vi "SMTP Email Alerts Engine.vi"(0 "Notifier Name":string, 11 "Ports (not used)":string[](array[string])) -> ()   [LabVIEW 2016]
uses:
  SMTP Email Alerts Type Defs/SMTP Email Alerts Notifier Type.ctl
  SMTP Email Alerts Type Defs/SMTP Email Alerts Actions.ctl
  <vilib>/smtpClient/Set Message Text.vi
  <vilib>/smtpClient/LabVIEWSMTPClient.lvlib
panel:
  out "Error":errorcluster
  in  "Quit":bool
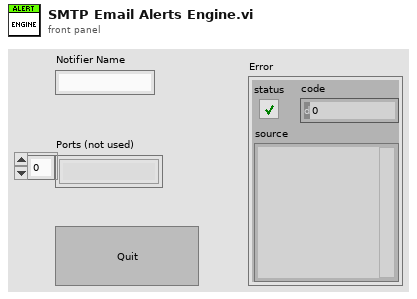
[diagram p1: front panel]
types:
  T1 = typedef "SMTP Email Alerts Notifier Type.ctl" = cluster{"Actions":T2, "Recipient":string, "Subject":string, "Message":string}
  T2 = typedef "SMTP Email Alerts Actions.ctl" = enum16{"Set Recipient", "Send Message", "Quit"}
  T3 = typedef "LabVIEWSMTPClient.lvlib/SmtpClientHandle.ctl" = refnum<k1>
  T4 = enum32{"Invalid", "Standard", "Closed", "Hidden", "Minimized", "Maximized"}
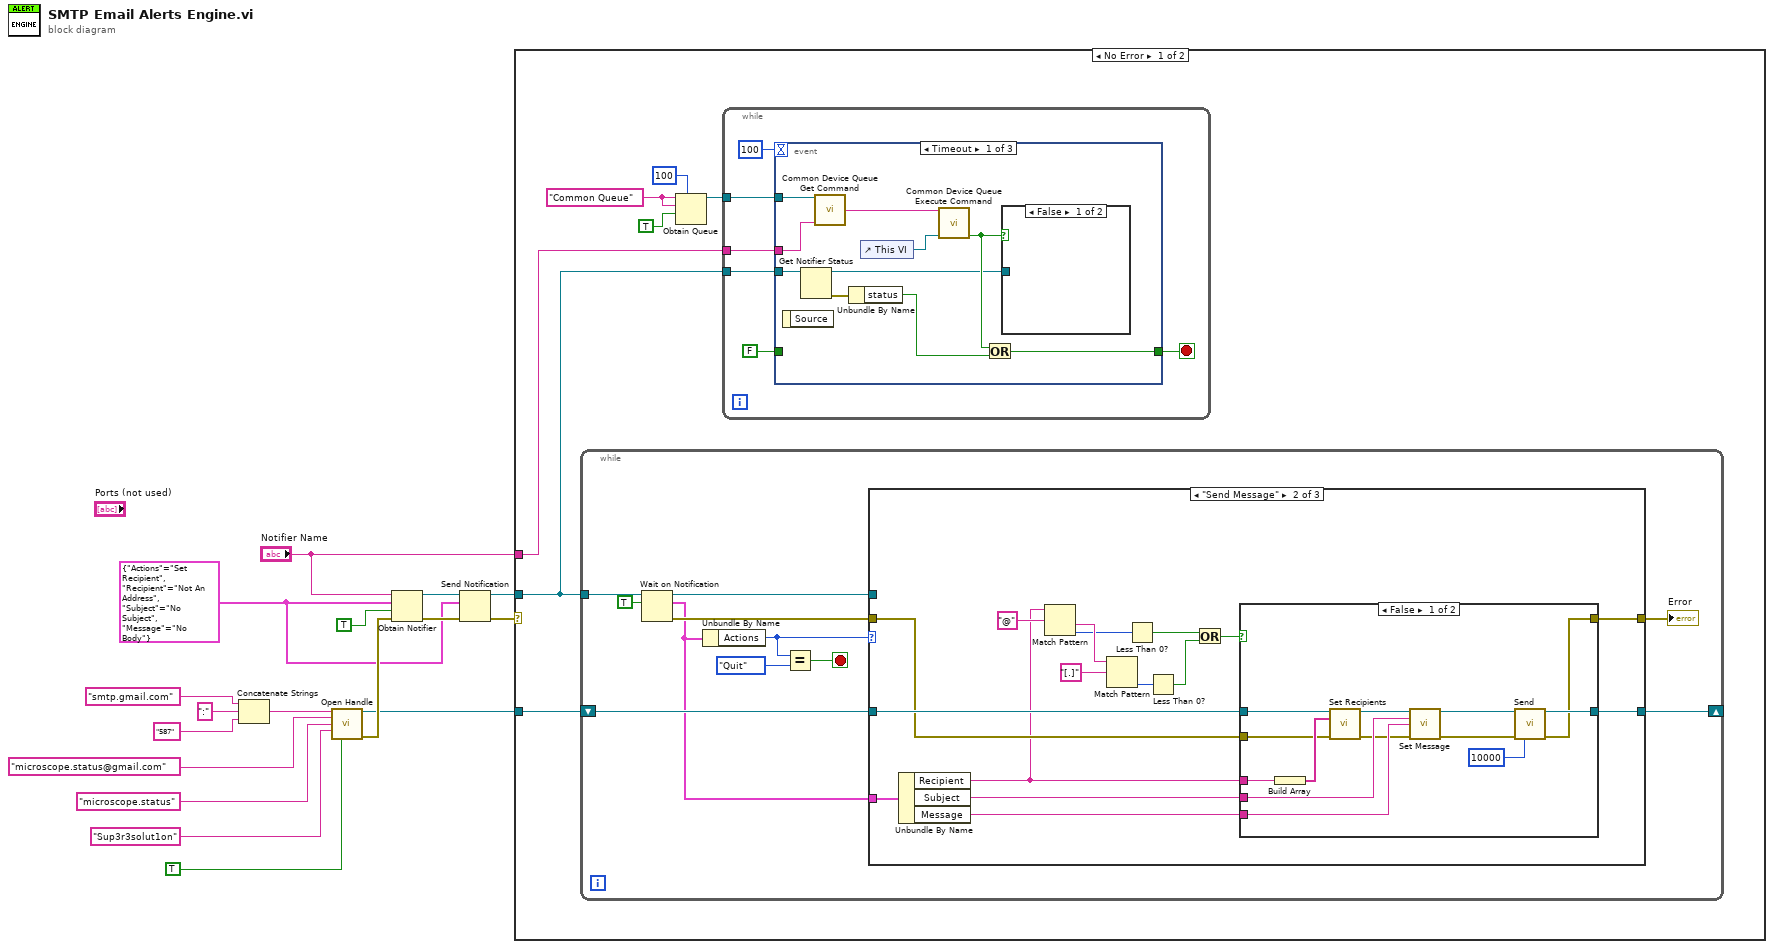
[diagram p0: block diagram]
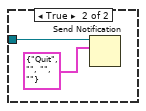
[diagram p2: hidden frame]
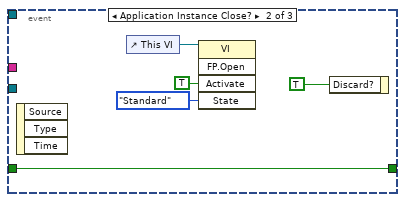
[diagram p3: hidden frame]
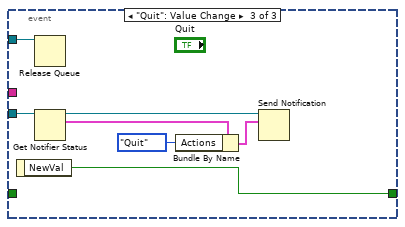
[diagram p4: hidden frame]
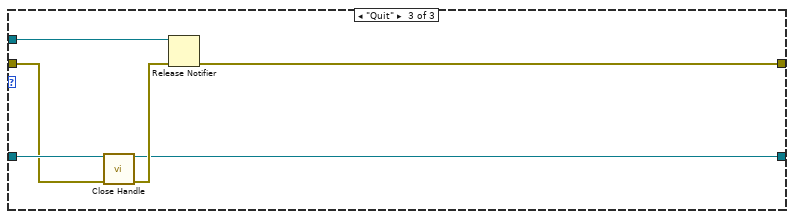
[diagram p7: hidden frame]
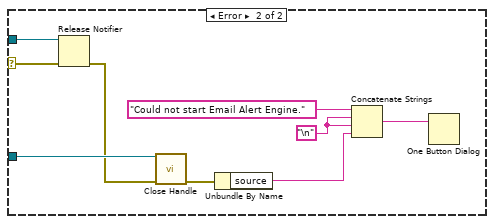
[diagram p8: hidden frame]
diagram:
  w1 = T1 {"Actions"=enum."Set Recipient", "Recipient"="Not An Address", "Subject"="No Subject", "Message"="No Body"} ("Message Info")
  n1 = Concatenate Strings("smtp.gmail.com" ("Outgoing Mail Server (SMTP)"), ":" ("string"), "587" ("Port")) -> (w13:string)
  n2 = call <vilib>:"Open Handle.vi"("server address"=w13, "from"="microscope.status@gmail.com" ("Sender's Email Address"), "username"="microscope.status" ("Username"), "password"="Sup3r3solut1on" ("Password"), "use TLS (false)"=TRUE ("Enable TLS")) -> ("handle out"=w8:T3, "error out"=w9:errorcluster)  [unwired: 9 in]
  n3 = Obtain Notifier(name (unnamed)="Notifier Name", notification data type=w1, create if not found? (T)=TRUE, error in (no error)=w9) -> (notifier out=w5:refnum<notifier>, error out=w3:errorcluster)  [unwired: 1 out]
  n4 = Send Notification(notification=w1, notifier=w5, error in (no error)=w3) -> (notifier out=w4:refnum<notifier>, error out=w2:errorcluster)
  n5 = case shown="No Error" w2 {
    selector: w2 -> [_ w111]
    tunnel: w4 -> [w19 w112]
    tunnel: w8 -> [w24 w113]
    tunnel: "Notifier Name" -> [w18 _]
    frame No Error {
      w20 = "Common Queue" ("Unique Notifier Name")
      n6 = while {
        tunnel: w19 -> [w65]
        shift-right: [w58] -> _
        shift-left: w24 -> [w59]
        stop <- w62 stop-if-true
        n7 = Wait on Notification(notifier=w65, ignore previous (F)=TRUE) -> (notifier out=w60:refnum<notifier>, notification=w56:T1, error out=w57:errorcluster)  [unwired: 2 in, 1 out]
        n8 = Unbundle By Name(w56) -> ("Actions"=w61:T2)
        n9 = Equal?(x=w61, y=SMTP_Email_Alerts_Actions."Quit") -> (x = y?=w62:bool)
        n10 = case shown="\"Send Message\"" w61 {
          tunnel: w60 -> [_ _ w103]
          tunnel: w59 -> [w66 w83 w102]
          tunnel: [w66 w81 w99] -> w58
          tunnel: w57 -> [w67 w78 w101]
          tunnel: w56 -> [_ w82 _]
          tunnel: [w67 w77 w100] -> w55
          frame Default {
          }
          frame "Send Message" {
            n11 = Unbundle By Name(w82) -> ("Recipient"=w68:string, "Subject"=w80:string, "Message"=w79:string)
            n12 = Match Pattern(string=w68, regular expression="@") -> (after substring=w76:string, offset past match=w73:i32)  [unwired: 1 in, 2 out]
            n13 = Match Pattern(string=w76, regular expression="[.]") -> (offset past match=w71:i32)  [unwired: 1 in, 3 out]
            n14 = Less Than 0?(x=w73) -> (x < 0?=w72:bool)
            n15 = Less Than 0?(x=w71) -> (x < 0?=w70:bool)
            n16 = Or(x=w72, y=w70) -> (x .or. y?=w69:bool)
            n17 = case shown="False" w69 {
              tunnel: w83 -> [w96 w98]
              tunnel: [w90 w98] -> w81
              tunnel: w80 -> [w89 _]
              tunnel: w79 -> [w88 _]
              tunnel: w78 -> [w86 w97]
              tunnel: [w85 w97] -> w77
              tunnel: w68 -> [w84 _]
              frame False {
                n18 = Build Array(w84) -> (w95:string[])
                n19 = call <vilib>:"Set Recipients.vi"("handle in"=w96, "to"=w95, "error in (no error)"=w86) -> ("handle out"=w91:T3, "error out"=w87:errorcluster)  [unwired: 11 in]
                n20 = call-poly <vilib>:"Set Message.vi"("handle in"=w91, "subject"=w89, "plain text message"=w88, "error in (no error)"=w87) -> ("handle out"=w93:T3, "error out"=w92:errorcluster)  [unwired: 10 in]
                n21 = call <vilib>:"Send.vi"("handle in"=w93, "error in (no error)"=w92, "timeout in ms (10000)"=10000 ("timeout in ms")) -> ("handle out"=w90:T3, "error out"=w85:errorcluster)  [unwired: 10 in, 1 out]
              }
              frame True {
              }
            }
          }
          frame "Quit" {
            n22 = call <vilib>:"Close Handle.vi"("handle in"=w102, "error in (no error)"=w101) -> ("handle out"=w99:T3, "error out"=w104:errorcluster)  [unwired: 12 in]
            n23 = Release Notifier(notifier=w103, error in (no error)=w104) -> (error out=w100:errorcluster)  [unwired: 1 in, 2 out]
          }
        }
        "Error" <- w55
      }
      n24 = Obtain Queue(max queue size (-1, unlimited)=100, name (unnamed)=w20, element data type=w20, create if not found? (T)=TRUE) -> (queue out=w23:refnum<queue>)  [unwired: 1 in, 2 out]
      n25 = while {
        tunnel: w23 -> [w30]
        tunnel: w19 -> [w27]
        tunnel: w18 -> [w25]
        stop <- w26 stop-if-true
        n26 = event shown="[0] Timeout" {
          selector: _ -> [_ _ _]
          dyn-events: _ -> [_ _ _]
          timeout: 100 -> [_ _ _]
          tunnel: w30 -> [w38 _ w49]
          tunnel: FALSE -> [_ w47 _]
          tunnel: w27 -> [w40 _ w50]
          tunnel: [w33 w47 w54] -> w26
          tunnel: w25 -> [w37 _ _]
          event Timeout {
            n27 = event-data() -> ()  [unwired: 1 in, 1 out]
            n28 = Get Notifier Status(notifier=w40) -> (notifier out=w31:refnum<notifier>, error out=w39:errorcluster)  [unwired: 1 in, 3 out]
            n29 = call "Common Device Queue Get Command.vi"("Common Queue"=w38, "Notifier Name"=w37) -> ("Command"=w36:string)  [unwired: 12 in, 1 out]
            n30 = Unbundle By Name(w39) -> ("status"=w34:bool)
            n31 = control-ref of="This VI"() -> (w35:refnum<vi>)
            n32 = call "Common Device Queue Execute Command.vi"("Common Command"=w36, "VI Refnum"=w35) -> ("Quit?"=w32:bool)  [unwired: 12 in, 1 out]
            n33 = Or(x=w32, y=w34) -> (x .or. y?=w33:bool)
            n34 = case shown="False" w32 {
              tunnel: w31 -> [_ w42]
              frame False {
              }
              frame True {
                n35 = Send Notification(notification=T1 {"Actions"=enum."Quit", "Recipient"="", "Subject"="", "Message"=""}, notifier=w42) -> ()  [unwired: 1 in, 2 out]
              }
            }
          }
          event Application Instance Close? {
            n36 = event-data() -> ()  [unwired: 1 in, 3 out]
            n37 = control-ref of="This VI"() -> (w44:refnum<vi>)
            n38 = invoke class="VI" method="FP.Open"(reference=w44, "Activate"=TRUE ("Activate?"), "State"=T4."Standard") -> ()  [unwired: 2 in, 5 out]
            n39 = event-data("Discard?"=TRUE) -> ()  [unwired: 1 in, 1 out]
          }
          event "Quit": Value Change {
            n40 = event-data() -> ("NewVal"=w54:bool)  [unwired: 1 in]
            n41 = Release Queue(queue=w49) -> ()  [unwired: 2 in, 3 out]
            n42 = Get Notifier Status(notifier=w50) -> (notifier out=w53:refnum<notifier>, current notification=w52:T1)  [unwired: 1 in, 3 out]
            n43 = Bundle By Name(cluster=w52, "Actions"=SMTP_Email_Alerts_Actions."Quit") -> (w51:T1)
            n44 = Send Notification(notification=w51, notifier=w53) -> ()  [unwired: 1 in, 2 out]
          }
        }
      }
    }
    frame Error {
      w107 = "\n"
      n45 = Release Notifier(notifier=w112, error in (no error)=w111) -> (error out=w110:errorcluster)  [unwired: 1 in, 2 out]
      n46 = call <vilib>:"Close Handle.vi"("handle in"=w113, "error in (no error)"=w110) -> ("error out"=w109:errorcluster)  [unwired: 12 in, 1 out]
      n47 = Unbundle By Name(w109) -> ("source"=w106:string)
      n48 = Concatenate Strings("Could not start Email Alert Engine.", w107, w107, w106) -> (w105:string)
      n49 = One Button Dialog(message=w105) -> ()  [unwired: 1 in, 1 out]
    }
  }
